vi "Autonomous Independent.vi"   [LabVIEW 2019]
doc: "This VI is called when autonomous begins, and will automatically be terminated when autonomous ends. You can carry out timed or sensor driven robot movement independently without needing to return to the caller."
uses:
  Robot Global Data.vi
  <vilib>/Rock Robotics/Network Tables/NT Read String.vi
  <vilib>/Rock Robotics/Network Tables/NT Write Numeric Array.vi
panel:
  # "Be sure to right-click and choose Data Operations>>Make Current Value default if you want to save the array values with the VI"
types:
  T1 = typedef "WPI_JoystickDevRef.ctl" = cluster{"Device":T2}
  T2 = typedef "WPI_JoystickDeviceEnum.ctl" = enum16{"USB 0", "USB 1", "USB 2", "USB 3", "USB 4", "USB 5"}
  T3 = typedef "WPI_ServoDeviceRef.ctl" = cluster{"DeviceStatus":errorcluster, "PWM Channel":T4, "DeadBand":T5}
  T4 = typedef "FPGA_DIOPWMChannel.ctl" = enum8{"PWM 0", "PWM 1", "PWM 2", "PWM 3", "PWM 4", "PWM 5", "PWM 6", "PWM 7", "PWM 8", "PWM 9", "PWM MXP 0", "PWM MXP 1", "PWM MXP 2", "PWM MXP 3", "PWM MXP 4", "PWM MXP 5", "PWM MXP 6", "PWM MXP 7", "PWM MXP 8", "PWM MXP 9", "Invalid"}
  T5 = typedef "WPI_PWMDeadband.ctl" = cluster{"Name":string, "maxPositivePwm":i32, "minPositivePwm":i32, "centerPwm":i32, "maxNegativePwm":i32, "minNegativePwm":i32, "angularRange":u16}
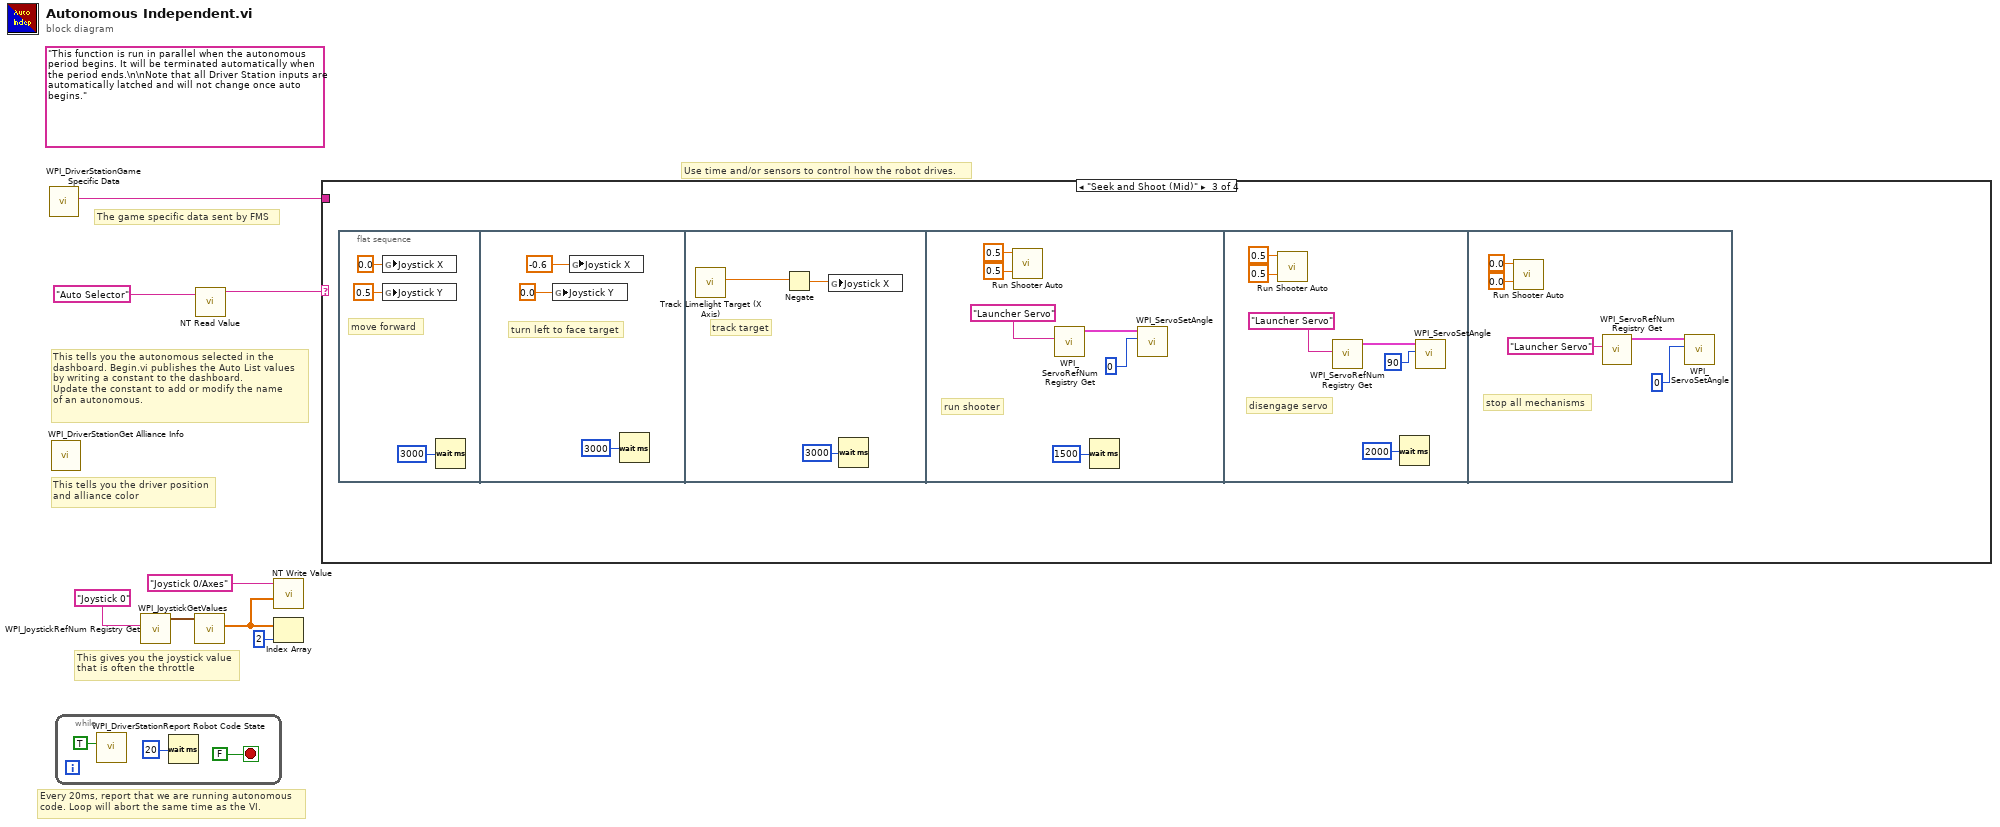
[diagram p0: block diagram]
diagram:
  (unwired) "This function is run in parallel when the autonomous period begins. It will be terminated automatically when the period ends.\n\nNote that all Driver Station inputs are automatically latched and will not change once auto begins."
  # "The game specific data sent by FMS"
  # "This tells you the autonomous selected in the \ndashboard. Begin.vi publishes the Auto List values\nby writing a constant to the dashboard.\nUpdate the constant to add or modify the name\nof an autonomous."
  # "Every 20ms, report that we are running autonomous\ncode. Loop will abort the same time as the VI."
  # "This gives you the joystick value\nthat is often the throttle"
  # "Use time and/or sensors to control how the robot drives."
  # "This tells you the driver position\nand alliance color"
  n1 = call <vilib>:"WPI_DriverStationGame Specific Data.vi"() -> ("Game Specific Data"=w1:string)  [unwired: 11 in]
  n2 = call <vilib>:"WPI_DriverStationGet Alliance Info.vi"() -> ()  [unwired: 12 out]
  n3 = while {
    stop <- FALSE stop-if-true
    n4 = call <vilib>:"WPI_DriverStationReport Robot Code State.vi"("Autonomous"=TRUE) -> ()  [unwired: 10 in, 1 out]
    n5 = Wait (ms)(milliseconds to wait=u32 20) -> ()  [unwired: 1 out]
  }
  n6 = call <vilib>:"WPI_JoystickRefNum Registry Get.vi"("refnum name"="Joystick 0") -> ("JoystickDevRef"=w7:T1)  [unwired: 1 in, 9 out]
  n7 = call <vilib>:"WPI_JoystickGetValues.vi"("JoystickDevRef"=w7) -> ("Axes"=w3:dbl[])  [unwired: 6 in, 4 out]
  n8 = call-poly <vilib>:"NT Read Value.vi"("Name"="Auto Selector") -> ("String"=w4:string)  [unwired: 9 in, 1 out]
  n9 = call-poly <vilib>:"NT Write Value.vi"("Numeric Array"=w3, "Name"="Joystick 0/Axes") -> ()  [unwired: 9 in, 1 out]
  n10 = Index Array(array=w3, index=2) -> ()  [unwired: 1 out]
  n11 = case shown="\"Seek and Shoot (Mid)\"" w4 {
    tunnel: w1 -> [_ _ _ _]
    frame Default {
      # "You can put your main auto here, or you can right-click on the case and make any\nother frame be the default case."
      # "This is the frame that will execute if no selection is made, or if it is not recognized"
    }
    frame "Seek and Shoot (L)" {
      n12 = flat-sequence {
        frame #0 {
        }
      }
    }
    frame "Seek and Shoot (Mid)" {
      n13 = flat-sequence {
        frame #0 {
          # "move forward"
          n14 = global write "Robot Global Data.vi" "Joystick X"(0.0 ("Joystick X")) -> ()
          n15 = global write "Robot Global Data.vi" "Joystick Y"(0.5 ("Joystick Y")) -> ()
          n16 = Wait (ms)(milliseconds to wait=u32 3000) -> ()  [unwired: 1 out]
        }
        frame #1 {
          # "turn left to face target"
          n17 = global write "Robot Global Data.vi" "Joystick Y"(0.0 ("Auto R")) -> ()
          n18 = global write "Robot Global Data.vi" "Joystick X"(-0.6 ("Auto L")) -> ()
          n19 = Wait (ms)(milliseconds to wait=u32 3000) -> ()  [unwired: 1 out]
        }
        frame #2 {
          # "track target"
          n20 = call "Track Limelight Target (X Axis).vi"() -> ("Joystick X"=w19:dbl)  [unwired: 11 in]
          n21 = Negate(x=w19) -> (-x=w18:dbl)
          n22 = global write "Robot Global Data.vi" "Joystick X"(w18) -> ()
          n23 = Wait (ms)(milliseconds to wait=u32 3000) -> ()  [unwired: 1 out]
        }
        frame #3 {
          # "run shooter"
          n24 = call "Run Shooter Auto.vi"("Bottom"=0.5, "Top"=0.5) -> ()  [unwired: 10 in]
          n25 = call <vilib>:"WPI_ServoRefNum Registry Get.vi"("refnum name"="Launcher Servo") -> ("ServoDeviceRef"=w23:T3)  [unwired: 9 in, 1 out]
          n26 = Wait (ms)(milliseconds to wait=u32 1500) -> ()  [unwired: 1 out]
          n27 = call <vilib>:"WPI_ServoSetAngle.vi"("Angle"=0, "ServoDeviceRef"=w23) -> ()  [unwired: 8 in, 2 out]
        }
        frame #4 {
          # "disengage servo"
          n28 = call "Run Shooter Auto.vi"("Bottom"=0.5, "Top"=0.5) -> ()  [unwired: 10 in]
          n29 = call <vilib>:"WPI_ServoRefNum Registry Get.vi"("refnum name"="Launcher Servo") -> ("ServoDeviceRef"=w29:T3)  [unwired: 9 in, 1 out]
          n30 = Wait (ms)(milliseconds to wait=u32 2000) -> ()  [unwired: 1 out]
          n31 = call <vilib>:"WPI_ServoSetAngle.vi"("Angle"=90, "ServoDeviceRef"=w29) -> ()  [unwired: 8 in, 2 out]
        }
        frame #5 {
          # "stop all mechanisms"
          n32 = call "Run Shooter Auto.vi"("Bottom"=0.0, "Top"=0.0) -> ()  [unwired: 10 in]
          n33 = call <vilib>:"WPI_ServoRefNum Registry Get.vi"("refnum name"="Launcher Servo") -> ("ServoDeviceRef"=w35:T3)  [unwired: 9 in, 1 out]
          n34 = call <vilib>:"WPI_ServoSetAngle.vi"("Angle"=0, "ServoDeviceRef"=w35) -> ()  [unwired: 8 in, 2 out]
        }
      }
    }
    frame "Seek and Shoot (R)" {
      n35 = flat-sequence {
        frame #0 {
        }
      }
    }
  }
